vi "Array (dbl) with nan replaced.vi"(11 "Data In":dbl[](array[numeric])) -> (1 "First Number":i32, 2 "'nan' filtered":i32, 3 "Filtered out NAN":dbl[](array[numeric]))   [LabVIEW 2013]
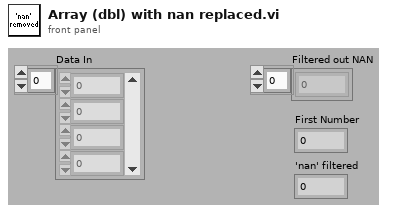
[diagram p1: front panel]
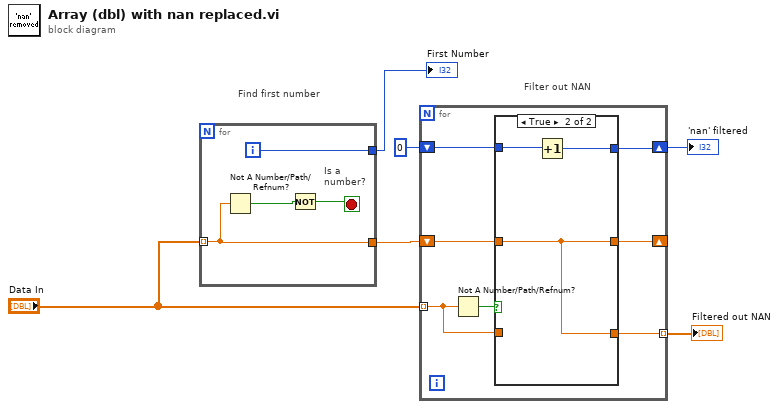
[diagram p0: block diagram]
diagram:
  # "Find first number"
  # "Filter out NAN"
  n1 = for {
    tunnel: "Data In" -> [w9] mode=indexing
    tunnel: [w9] -> w4
    tunnel: [w7] -> w3
    i -> [w7]
    stop <- w8 stop-if-true
    # "Is a \nnumber?"
    n2 = Not A Number/Path/Refnum?(number/path/refnum=w9) -> (NaN/Path/Refnum?=w10:bool)
    n3 = Not(x=w10) -> (.not. x?=w8:bool)
  }
  "First Number" <- w3
  n4 = for {
    tunnel: "Data In" -> [w15] mode=indexing
    shift-right: [w14] -> _
    shift-left: w4 -> [w16]
    tunnel: [w13] -> w5 mode=indexing
    shift-right: [w11] -> w2
    shift-left: 0 ("'nan' filtered") -> [w12]
    n5 = Not A Number/Path/Refnum?(number/path/refnum=w15) -> (NaN/Path/Refnum?=w17:bool)
    n6 = case shown="True" w17 {
      tunnel: w16 -> [_ w22]
      tunnel: [w19 w22] -> w13
      tunnel: w15 -> [w19 _]
      tunnel: [w19 w22] -> w14
      tunnel: w12 -> [w18 w21]
      tunnel: [w18 w20] -> w11
      frame False {
      }
      frame True {
        n7 = Increment(x=w21) -> (x+1=w20:i32)
      }
    }
  }
  "Filtered out NAN" <- w5
  "'nan' filtered" <- w2
